vi "Periodic Tasks.vi"(8 "error in":errorcluster) -> ()   [LabVIEW 2016]
doc: "This VI runs in parallel to other tasks. It can contain as many user-defined periodic loops as you need. These can carry out PID or other sorts of timed response."
uses:
  <vilib>/Rock Robotics/Network Tables/NT Write Numeric Array.vi
panel:
  in  "Front Left":dbl(knob)=0.33686582702293943 scale=-0.5..0.5
  in  "Front right":dbl(knob)=-0.007019271019562789 scale=-0.5..0.5
  in  "Back left":dbl(knob)=0.21563214632755767 scale=-0.5..0.5
  in  "Back right":dbl(knob)=0.2726030483023637 scale=-0.5..0.5
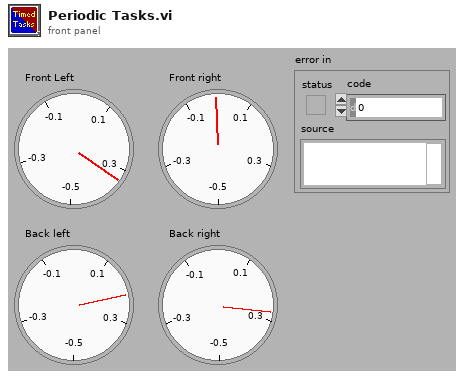
[diagram p1: front panel]
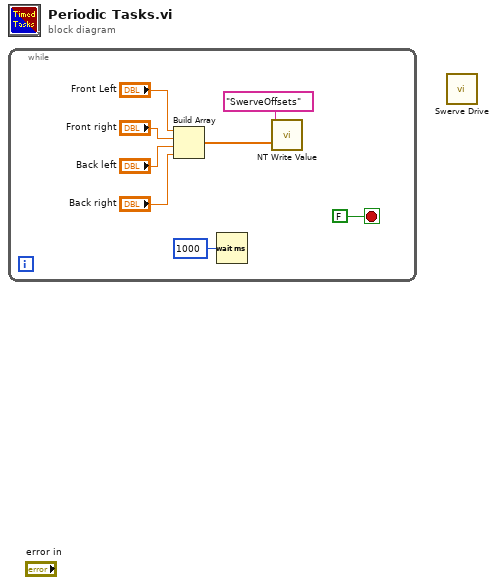
[diagram p0: block diagram]
diagram:
  n1 = while {
    stop <- FALSE stop-if-true
    n2 = Build Array("Front Left", "Front right", "Back left", "Back right") -> (w4:dbl[])
    n3 = Wait (ms)(milliseconds to wait=u32 1000) -> ()  [unwired: 1 out]
    n4 = call-poly <vilib>:"NT Write Value.vi"("Numeric Array"=w4, "Name"="SwerveOffsets") -> ()  [unwired: 9 in, 1 out]
  }
  n5 = call "Swerve Drive.vi"() -> ()  [unwired: 16 in]
